vi "Set Operations Queue.vi"(8 "error in (no error)":errorcluster, 10 "Data":variant, 11 "Command":string) -> (0 "error out":errorcluster)   [LabVIEW 2014]
uses:
  Controls/Data Queue.ctl
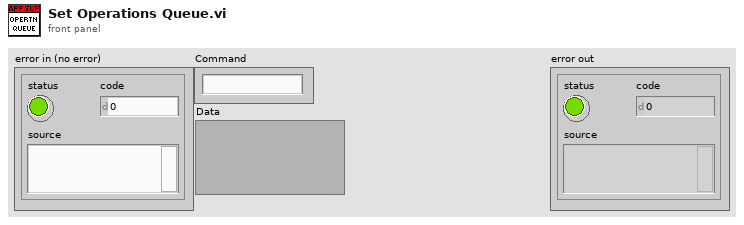
[diagram p1: front panel]
types:
  T1 = typedef "Data Queue.ctl" = cluster{"Command":string, "Data":variant}
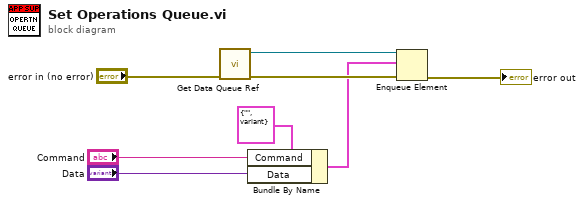
[diagram p0: block diagram]
diagram:
  n1 = call "Get Data Queue Ref.vi"("error in (no error)"="error in (no error)") -> ("error out"=w6:errorcluster, "Ground Station Operations Queue Ref"=w7:refnum<queue>)  [unwired: 9 in]
  n2 = Bundle By Name(cluster=T1 {"Command"="", "Data"=variant} ("element"), "Command"="Command", "Data"="Data") -> (w3:T1)
  n3 = Enqueue Element(queue=w7, element=w3, error in (no error)=w6) -> (error out=→"error out":errorcluster)  [unwired: 1 in, 2 out]
